vi "DeviceQuery.vi"(4 "error in (no error)":errorcluster, 5 "Command":string, 6 "DeviceKey In":string, 7 "CmdLib In":refnum<k24>) -> (0 "error out":errorcluster, 1 "Response":string, 2 "DeviceKey Out":string, 3 "CmdLib Out":refnum<k24>)   [LabVIEW 2013]
uses:
  C:/Users/Saffmanlab/Documents/git/CsPyController/labview/cesium_controller/PicoMotor/NewFocus8742/CmdLib.dll
  CmdLib.dll
panel:
  in  "value":string
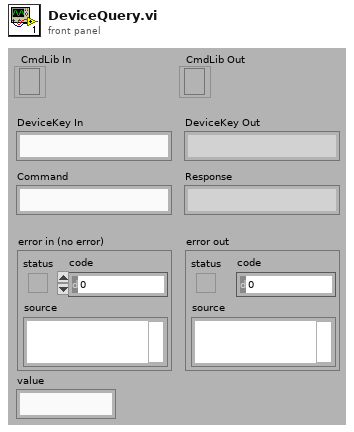
[diagram p1: front panel]
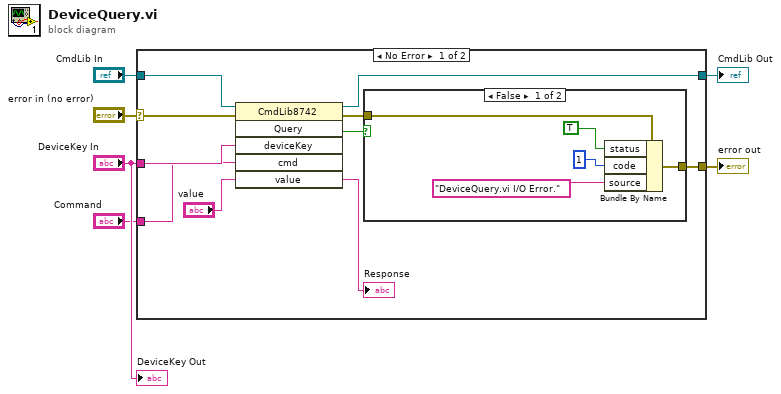
[diagram p0: block diagram]
diagram:
  n1 = case shown="No Error" "error in (no error)" {
    selector: "error in (no error)" -> [w13 w24]
    tunnel: "CmdLib In" -> [w16 w23]
    tunnel: [w15 w23] -> w5
    tunnel: "DeviceKey In" -> [w14 _]
    tunnel: [w10 w24] -> w2
    tunnel: "Command" -> [w7 _]
    frame No Error {
      n2 = invoke class="CmdLib8742" method="Query"(reference=w16, error in=w13, "deviceKey"=w14, "cmd"=w7, "value"="value") -> (reference out=w15:refnum<k24>, error out=w11:errorcluster, "Query"=w12:bool, "value"=→"Response":string)  [unwired: 1 in, 2 out]
      n3 = case shown="False" w12 {
        tunnel: w11 -> [w19 w22]
        tunnel: [w18 w22] -> w10
        frame False {
          n4 = Bundle By Name(cluster=w19, "status"=TRUE, "code"=1, "source"="DeviceQuery.vi I/O Error.") -> (w18:errorcluster)
        }
        frame True {
        }
      }
    }
    frame Error {
    }
  }
  "CmdLib Out" <- w5
  "error out" <- w2
  "DeviceKey Out" <- "DeviceKey In"
